vi "globals.vi"() -> ()   [LabVIEW 2017]
uses:
  Types/ExperimentGrp.ctl
  Types/SystemEventDataStruct.ctl
panel:
  out "GlobalInvoke":refnum<user-event>
  out "GlobalInvokeByCategoryCollection":variant
  out "GlobalInvoke Event Registration Refnum":refnum<event-registration>
  out "ButtonPressed":bool
  out "AvailableExperiments":T1[](array[typedef])
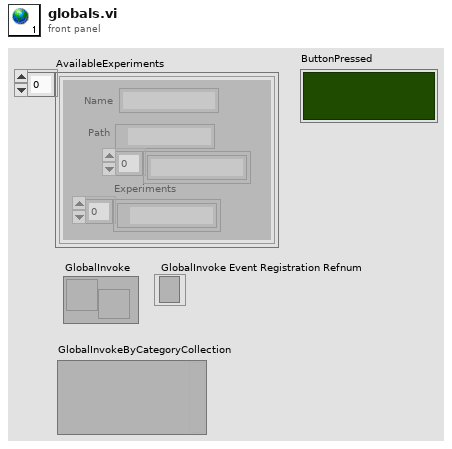
[diagram p1: front panel]
types:
  T1 = typedef "ExperimentGrp.ctl" = cluster{"Path":path, "Experiments":path[], "Name":string, "Experiment Names":string[]}
diagram:
